vi "Write ThisVI.vi"(8 "error in (no error)":errorcluster, 10 "ThisVI":refnum<vi>, 11 "Generator in":refnum<class "Generator.lvclass">) -> (0 "error out":errorcluster, 3 "Generator out":refnum<class "Generator.lvclass">)   [LabVIEW 2014, in "Generator.lvlib" / "Generator.lvclass"]
uses:
  Generator.lvclass
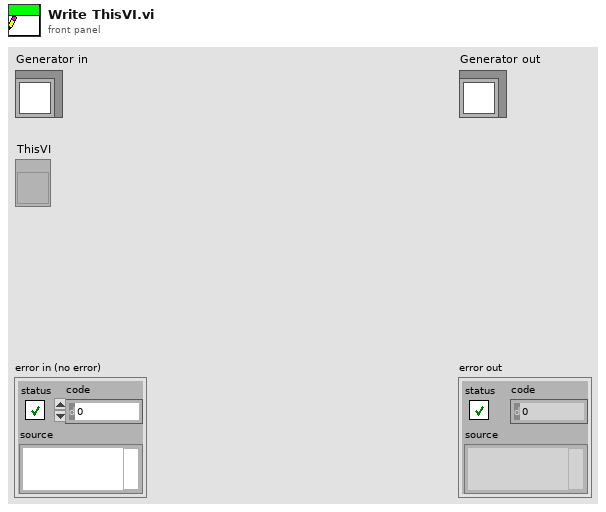
[diagram p1: front panel]
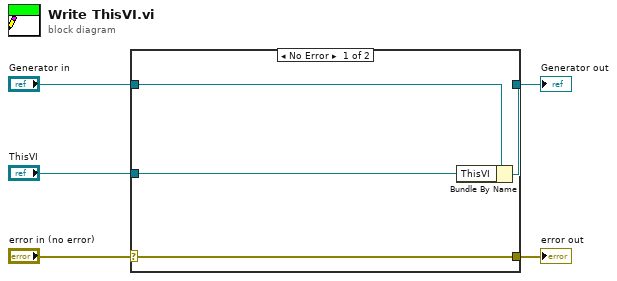
[diagram p0: block diagram]
diagram:
  n1 = case shown="No Error" "error in (no error)" {
    selector: "error in (no error)" -> [w9 w10]
    tunnel: [w9 w10] -> w4
    tunnel: [w7 w11] -> w2
    tunnel: "Generator in" -> [w8 w11]
    tunnel: "ThisVI" -> [w6 _]
    frame No Error {
      n2 = Bundle By Name(cluster=w8, "ThisVI"=w6) -> (w7:refnum<class "Generator.lvclass">)
    }
    frame Error {
    }
  }
  "error out" <- w4
  "Generator out" <- w2
